vi "Obtain Module Registred Broadcast.vi"(7 "Config":refnum<class "TAF Proj Config.lvclass">, 8 "error in":errorcluster, 11 "VI References":refnum<vi>[](array[refnum])) -> (0 "error out":errorcluster, 3 "Registred Broadcast":T1[](array[typedef]))   [LabVIEW 2021, in "TAF Proj Document Type.lvlib" / "Project Parser.lvlib"]
uses:
  <vilib>/Wovalab/AntiDoc/Document Type/Add-ons/LabVIEW TAF Project/Project Parser/Project Parser.lvlib
  <vilib>/Wovalab/AntiDoc/Document Type/Add-ons/LabVIEW TAF Project/Project Parser/Module Fonctions--cluster.ctl
  <vilib>/Wovalab/AntiDoc/Document Type/Add-ons/LabVIEW TAF Project/TAF Proj Config/TAF Proj Config.lvclass
  <vilib>/Wovalab/AntiDoc/Document Type/Add-ons/LabVIEW TAF Project/Project Parser/Module Fonctions--enum.ctl
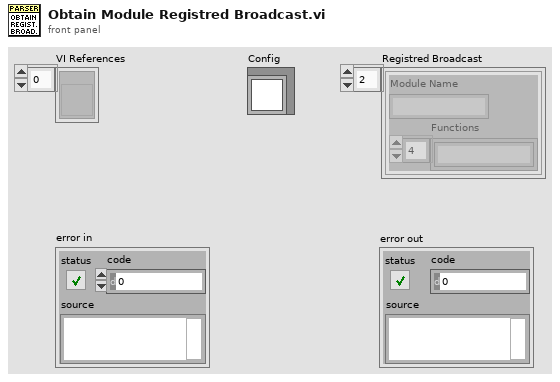
[diagram p1: front panel]
types:
  T1 = typedef "TAF Proj Document Type.lvlib/Project Parser.lvlib/Module Fonctions--cluster.ctl" = cluster{"Module Name":string, "Functions":string[]}
  T2 = typedef "TAF Proj Document Type.lvlib/Project Parser.lvlib/Module Fonctions--enum.ctl" = enum16{"Event Registration", "Request"}
  T3 = typedef "TAF Proj Document Type.lvlib/Project Parser.lvlib/User Event Info.ctl" = cluster{"Vi Name":string, "User Event Names":string[]}
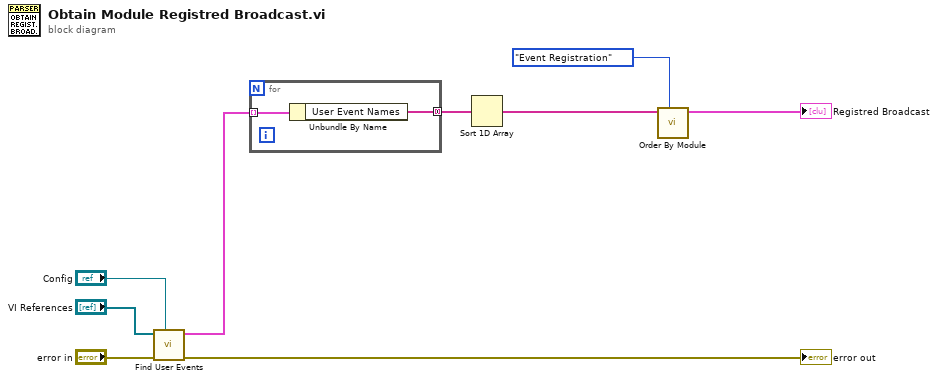
[diagram p0: block diagram]
diagram:
  n1 = call <vilib>:"Find User Events.vi"("Config"="Config", "error in"="error in", "VI References"="VI References") -> ("error out"=→"error out":errorcluster, "User Event  Info"=w3:T3[])  [unwired: 7 in]
  n2 = for {
    tunnel: w3 -> [w11] mode=indexing
    tunnel: [w10] -> w5 mode=concatenating
    n3 = Unbundle By Name(w11) -> ("User Event Names"=w10:string[])
  }
  n4 = Sort 1D Array(array=w5) -> (sorted array=w2:string[])
  n5 = call <vilib>:"Order By Module.vi"("Mode"=Module_Fonctions--enum."Event Registration", "Functions"=w2) -> ("Functions by Module"=→"Registred Broadcast":T1[])  [unwired: 9 in]
